vi "Stop Core.vi"(10 "final error code":i32, 11 "CS++Motor in":refnum<class "CS++Motor.lvclass">) -> (3 "CS++Motor out":refnum<class "CS++Motor.lvclass">)   [LabVIEW 2015, in "CS++Motor.lvlib" / "CS++Motor.lvclass"]
doc: "(<B>Filename</B>: Actor Framework.lvlib:Actor.lvclass:Stop Core.vi)\n\nDefines what the actor does before it stops. Use the <B>final error code</B> input to determine whether the actor shut down in response to an error.\n\nBy default, this method does nothing. A descendant class may override it to define behavior, such as shutting down any processes the actor initiated in its override of the Actor Core method."
uses:
  CS++Motor.lvclass
  CS++Motor.lvclass/CS++Motor.ctl
  CSPP_Core/Actors/CS++DeviceActor/CS++DeviceActor.lvclass
  CSPP_Core/Classes/CS++ProcessVariables/PVConnection/PVConnection.lvclass
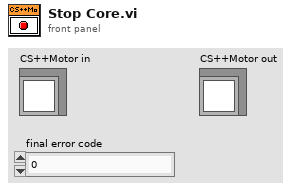
[diagram p1: front panel]
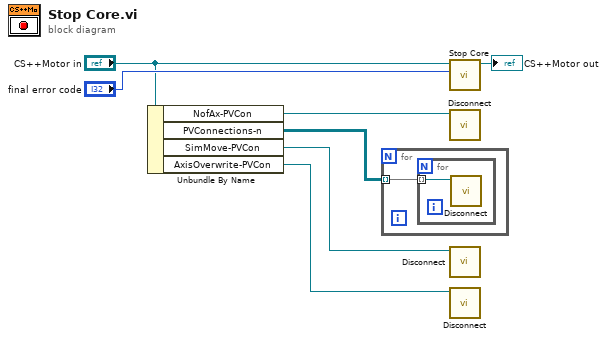
[diagram p0: block diagram]
diagram:
  n1 = Unbundle By Name("CS++Motor in") -> ("NofAx-PVCon"=w4:refnum<class "PVConnection.lvclass">, "PVConnections-n"=w3:refnum<class "PVConnection.lvclass">[][], "SimMove-PVCon"=w2:refnum<class "PVConnection.lvclass">, "AxisOverwrite-PVCon"=w1:refnum<class "PVConnection.lvclass">)
  n2 = for {
    tunnel: w3 -> [w8] mode=indexing
    n3 = for {
      tunnel: w8 -> [w9] mode=indexing
      n4 = call "Disconnect.vi"("PVConnection in"=w9) -> ()  [unwired: 9 in, 2 out]
    }
  }
  n5 = call-parent "Stop Core.vi"("final error code"="final error code", "CS++DeviceActor in"="CS++Motor in") -> ("CS++DeviceActor out"=→"CS++Motor out":refnum<class "CS++Motor.lvclass">)  [unwired: 9 in]
  n6 = call "Disconnect.vi"("PVConnection in"=w4) -> ()  [unwired: 9 in, 2 out]
  n7 = call "Disconnect.vi"("PVConnection in"=w2) -> ()  [unwired: 9 in, 2 out]
  n8 = call "Disconnect.vi"("PVConnection in"=w1) -> ()  [unwired: 9 in, 2 out]
